vi "Launch NIVS and get Ref.vi"(8 "error in (no error)":errorcluster) -> (0 "error out":errorcluster, 3 "WorkspaceManager":T1)   [LabVIEW 2011]
uses:
  <vilib>/NI Veristand/Execution/Workspace/WorkspaceAPI.ctl
  NationalInstruments.VeriStand.ClientAPI
  <vilib>/registry/registry.llb/Registry SAM.ctl
  <vilib>/registry/registry.llb/Read Registry Value Simple STR.vi
  <vilib>/NI Veristand/Execution/Workspace/NI_VS Workspace ExecutionAPI.lvlib
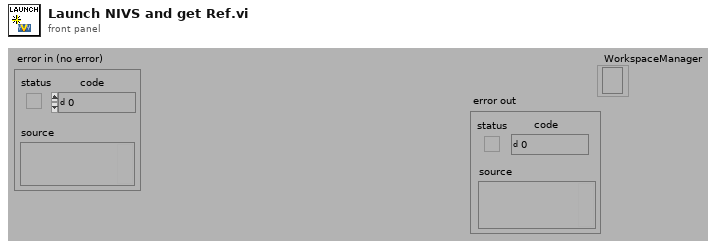
[diagram p1: front panel]
types:
  T1 = typedef "NI_VS Workspace ExecutionAPI.lvlib/WorkspaceAPI.ctl" = refnum<k24>
  T2 = typedef "Registry SAM.ctl" = enum32{"KEY_QUERY_VALUE", "KEY_SET_VALUE", "KEY_CREATE_SUB_KEY", "KEY_ENUMERATE_SUB_KEYS", "KEY_NOTIFY", "KEY_CREATE_LINK", "KEY_READ", "KEY_WRITE", "KEY_ALL_ACCESS", "KEY_READ | KEY_WRITE"}
  T3 = typedef "Registry refnum.ctl" = refnum<k1>
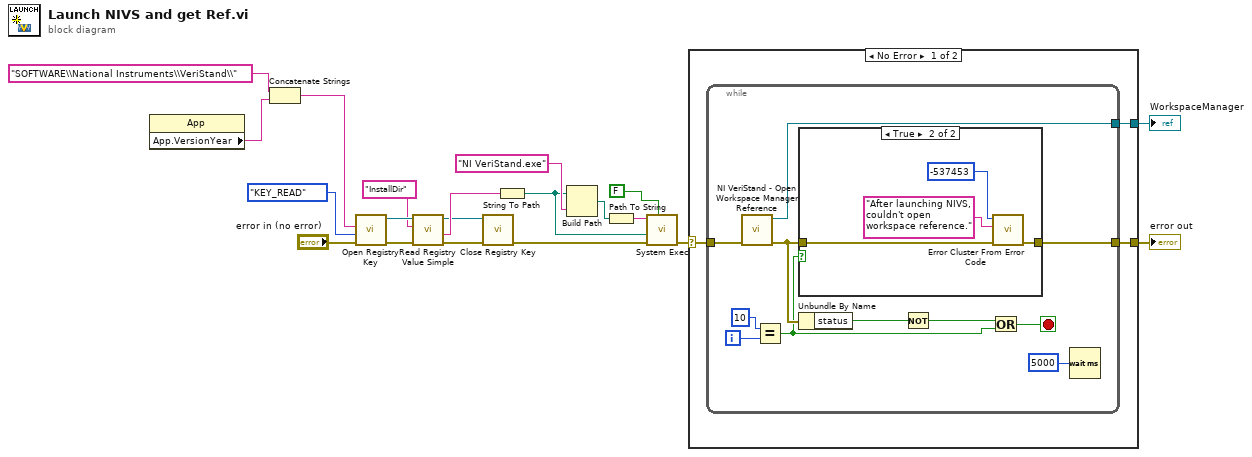
[diagram p0: block diagram]
diagram:
  n1 = property class="App"() -> ("App.VersionYear"=w2:string)  [unwired: 2 in, 2 out]
  n2 = Concatenate Strings("SOFTWARE\\National Instruments\\VeriStand\\" ("subkey"), w2) -> (w3:string)
  n3 = call <vilib>:"Open Registry Key.vi"("error in (no error)"="error in (no error)", "security access mask (KEY_READ | KEY_WRITE)"=Registry_SAM."KEY_READ", "subkey"=w3) -> ("error out"=w18:errorcluster, "refnum out"=w17:T3)  [unwired: 7 in]
  n4 = call-poly <vilib>:"Read Registry Value Simple.vi"("error in (no error)"=w18, "value"="InstallDir", "refnum"=w17) -> ("error out"=w13:errorcluster, "String/Binary data"=w15:string, "refnum out"=w12:T3)  [unwired: 3 in, 1 out]
  n5 = call <vilib>:"Close Registry Key.vi"("error in (no error)"=w13, "refnum"=w12) -> ("error out"=w11:errorcluster)  [unwired: 5 in]
  n6 = String To Path(string=w15) -> (path=w8:path)
  n7 = Build Path(base path=w8, name or relative path="NI VeriStand.exe") -> (appended path=w10:path)
  n8 = Path To String(path=w10) -> (string=w9:string)
  n9 = call <vilib>:"System Exec.vi"("wait until completion? (T)"=FALSE, "error in (no error)"=w11, "working directory"=w8, "command line"=w9) -> ("error out"=w6:errorcluster)  [unwired: 4 in, 3 out]
  n10 = case shown="No Error" w6 {
    selector: w6 -> [w23 w40]
    tunnel: [w22 w40] -> w5
    tunnel: [w21 _] -> w4
    frame No Error {
      n11 = while {
        tunnel: [w29] -> w21
        tunnel: w23 -> [w30]
        tunnel: [w31] -> w22
        i -> [w33]
        stop <- w24 stop-if-true
        n12 = call <vilib>:"NI VeriStand - Open Workspace Manager Reference.vi"("error in (no error)"=w30) -> ("error out"=w28:errorcluster, "WorkspaceManager"=w29:T1)  [unwired: 9 in]
        n13 = Equal?(x=10, y=w33) -> (x = y?=w25:bool)
        n14 = case shown="True" w25 {
          tunnel: [w35 w38] -> w31
          tunnel: w28 -> [w35 w39]
          frame False {
          }
          frame True {
            n15 = call <vilib>:"Error Cluster From Error Code.vi"("error in (no error)"=w39, "error message (\"\")"="After launching NIVS, couldn't open workspace reference." ("error message (\"\")"), "error code (0)"=-537453) -> ("error out"=w38:errorcluster)  [unwired: 6 in]
          }
        }
        n16 = Unbundle By Name(w28) -> ("status"=w27:bool)
        n17 = Not(x=w27) -> (.not. x?=w26:bool)
        n18 = Or(x=w26, y=w25) -> (x .or. y?=w24:bool)
        n19 = Wait (ms)(milliseconds to wait=u32 5000) -> ()  [unwired: 1 out]
      }
    }
    frame Error {
    }
  }
  "error out" <- w5
  "WorkspaceManager" <- w4
